vi "all_vis.vi"(8 "error in":errorcluster, 9 "try sorting first (fails if cycles found)?":bool, 11 "HierarchyGraph in":refnum<class "HierarchyGraph.lvclass">) -> (0 "error out":errorcluster, 1 "VIs":refnum<class "HierarchyNode.lvclass">[](array[class]), 3 "HierarchyGraph out":refnum<class "HierarchyGraph.lvclass">)   [LabVIEW 2020, in "vi-hierarchy.lvlib" / "HierarchyGraph.lvclass"]
uses:
  HierarchyGraph.lvclass
  C:/Projects/labview-project-load-tools/source/submodules/graph-api-labview/source/api/Graph/Graph.lvclass
  C:/Projects/labview-project-load-tools/source/submodules/graph-api-labview/source/api/DiGraph/DiGraph.lvclass
  VINode/HierarchyNode.lvclass
  api/Node/Node.lvclass
  api/Graph/Graph.lvclass
  api/DiGraph/DiGraph.lvclass
panel:
  out "exec time (s)":dbl
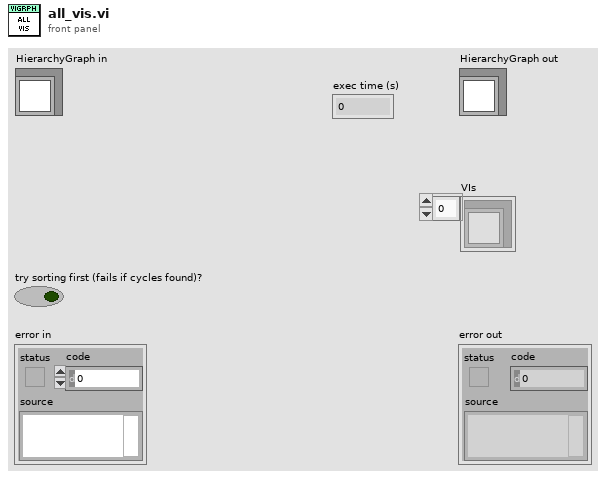
[diagram p1: front panel]
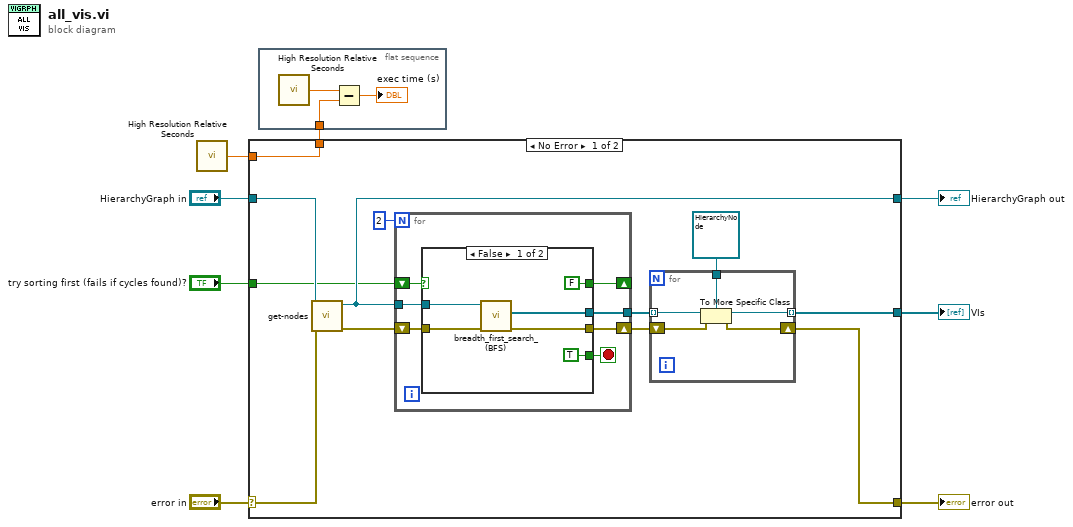
[diagram p0: block diagram]
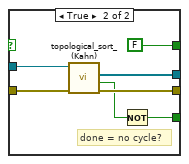
[diagram p2: hidden frame]
diagram:
  n1 = call <vilib>:"High Resolution Relative Seconds.vi"() -> ("relative seconds"=w2:dbl)
  n2 = case shown="No Error" "error in" {
    selector: "error in" -> [w19 w48]
    tunnel: [w16 w48] -> w7
    tunnel: [w15 w47] -> w5
    tunnel: "HierarchyGraph in" -> [w20 w47]
    tunnel: [w17 _] -> w4
    tunnel: "try sorting first (fails if cycles found)?" -> [w11 _]
    tunnel: [w9 w46] -> w1
    tunnel: w2 -> [w9 w46]
    frame No Error {
      n3 = call "get-nodes.vi"("error in (no error)"=w19, "Graph in"=w20) -> ("error out"=w14:errorcluster, "Graph out"=w15:refnum<class "HierarchyGraph.lvclass">)  [unwired: 7 in, 1 out]
      n4 = for {
        N: 2 -> [_]
        tunnel: w15 -> [w27]
        tunnel: [w24] -> w12
        shift-right: [w25] -> w13
        shift-left: w14 -> [w26]
        shift-right: [w21] -> _
        shift-left: w11 -> [w23]
        stop <- w22 stop-if-true
        n5 = case shown="False" w23 {
          tunnel: w27 -> [w30 w40]
          tunnel: w26 -> [w33 w39]
          tunnel: [w32 w38] -> w25
          tunnel: [w31 w37] -> w24
          tunnel: [TRUE w34] -> w22
          tunnel: [FALSE FALSE] -> w21
          frame False {
            n6 = call "breadth_first_search_(BFS).vi"("error in (no error)"=w33, "DiGraph in"=w30) -> ("error out"=w32:errorcluster, "nodes (by visit order)"=w31:refnum<class "Node.lvclass">[])  [unwired: 8 in]
          }
          frame True {
            # "done = no cycle?"
            n7 = call "topological_sort_(Kahn).vi"("error in (no error)"=w39, "DiGraph in"=w40) -> ("error out"=w38:errorcluster, "cycle detected"=w35:bool, "nodes (sorted)"=w37:refnum<class "Node.lvclass">[])  [unwired: 7 in]
            n8 = Not(x=w35) -> (.not. x?=w34:bool)
          }
        }
      }
      n9 = for {
        tunnel: w12 -> [w44] mode=indexing
        tunnel: refnum<class "HierarchyNode.lvclass"> refnum ("vi-hierarchy.lvlib:HierarchyNode.lvclass") -> [w45]
        tunnel: [w43] -> w17 mode=indexing
        shift-right: [w41] -> w16
        shift-left: w13 -> [w42]
        n10 = To More Specific Class(target class=w45, reference=w44, error in=w42) -> (specific class reference=w43:refnum<class "HierarchyNode.lvclass">, error out=w41:errorcluster)
      }
    }
    frame Error {
    }
  }
  "error out" <- w7
  "HierarchyGraph out" <- w5
  "VIs" <- w4
  n11 = flat-sequence {
    tunnel: w1 -> [w50]
    frame #0 {
      n12 = call <vilib>:"High Resolution Relative Seconds.vi"() -> ("relative seconds"=w51:dbl)
      n13 = Subtract(x=w51, y=w50) -> (x-y=→"exec time (s)":dbl)
    }
  }
